vi "term_op.vi"() -> ()   [LabVIEW 2020]
panel:
  out "Boolean 2":bool caption="LED 1"
  out "Boolean":bool caption="LED 2"
  out "led 2":dbl
  out "led 1":dbl
  out "Waveform Chart":dynamicdata(graph)
  out "Numeric 7":dbl
  out "Numeric 6":dbl
  out "Numeric 5":dbl
  out "Numeric 4":dbl
  out "Numeric 3":dbl
  out "Numeric 2":dbl
  out "Numeric":dbl
  in  "stop":bool
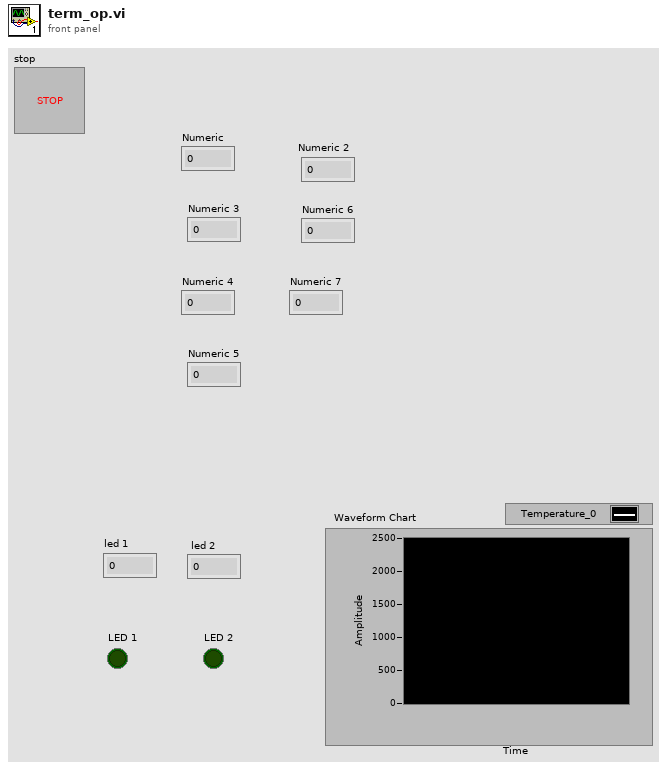
[diagram p1: front panel]
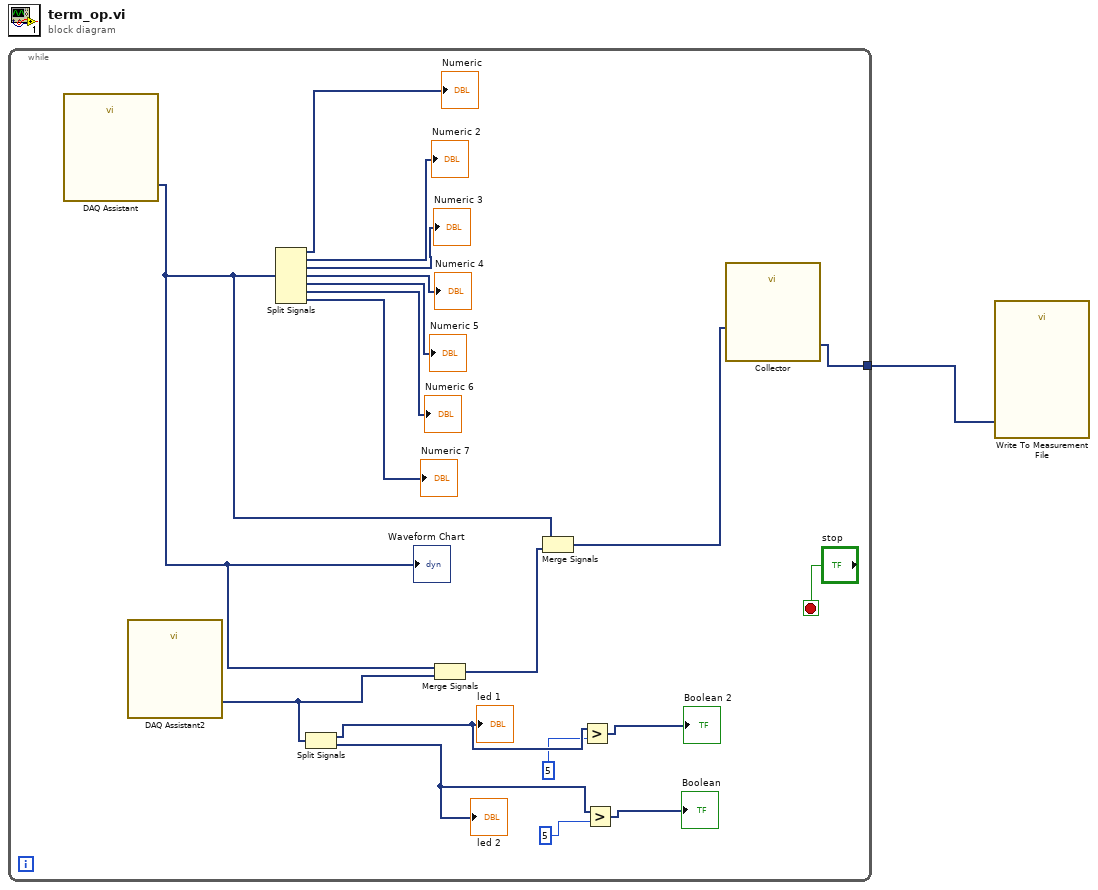
[diagram p0: block diagram]
diagram:
  n1 = while {
    tunnel: [w12] -> w1
    stop <- "stop" stop-if-true
    n2 = call "DAQ Assistant"() -> ("data"=w11:dynamicdata)  [unwired: 16 in, 3 out]
    "Waveform Chart" <- w11
    n3 = call "DAQ Assistant2"() -> ("data"=w8:dynamicdata)  [unwired: 17 in, 2 out]
    n4 = Split Signals(w11) -> (→"Numeric":dynamicdata, →"Numeric 2":dynamicdata, →"Numeric 3":dynamicdata, →"Numeric 4":dynamicdata, →"Numeric 5":dynamicdata, →"Numeric 6":dynamicdata, →"Numeric 7":dynamicdata)  [unwired: 7 in]
    n5 = Split Signals(w8) -> (w7:dynamicdata, w6:dynamicdata)  [unwired: 2 in]
    "led 1" <- w7
    "led 2" <- w6
    n6 = Merge Signals(w11, w8) -> (w9:dynamicdata)
    n7 = Merge Signals(w11, w9) -> (w10:dynamicdata)
    n8 = Greater?(x=w7, y=5) -> (0:→"Boolean 2":dynamicdata)
    n9 = Greater?(x=w6, y=5) -> (0:→"Boolean":dynamicdata)
    n10 = call "Collector"("Signals"=w10) -> ("Collected Signals"=w12:dynamicdata)  [unwired: 9 in, 1 out]
  }
  n11 = call "Write To Measurement File"("Signals"=w1) -> ()  [unwired: 16 in, 3 out]
